vi "02_VI_DAC.vi"() -> ()   [LabVIEW 2017]
doc: "This VI illustrates how to programmatically clear different types of charts. Charts can accept a single point at a time or multiple points at a time. The charts are cleared by writing empty arrays to the History Data property node."
panel:
  out "Waveform Chart (Multiple Plots)":cluster{dbl, dbl}(graph)
  in  "Clear":bool
  out "Waveform Chart":dbl(graph)
  in  "Stop":bool
  # "Overview: Demonstrates how to programmatically clear the contents of Waveform Charts.\nInstructions:\n1. Run the VI.\n2. Click Clear to clear the contents of the charts.\n3. Click Stop to stop the VI."
  # "While the VI is running, you can right-click a chart and select Clear Chart to interactively clear the contents of the chart."
  # "Un DAC genera 2 formas de Onda! :)"
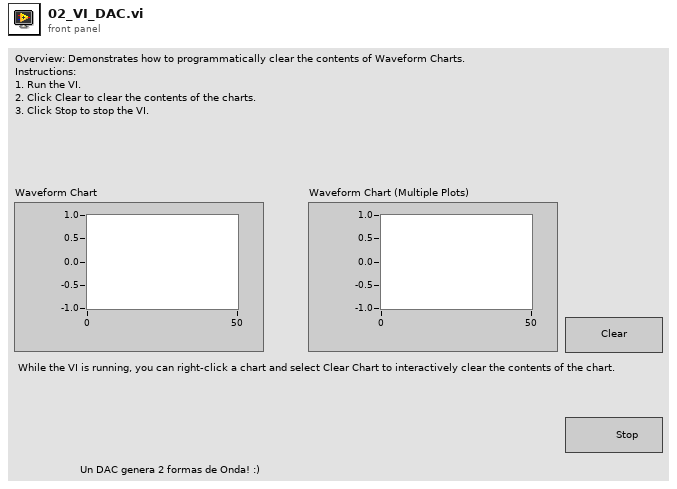
[diagram p1: front panel]
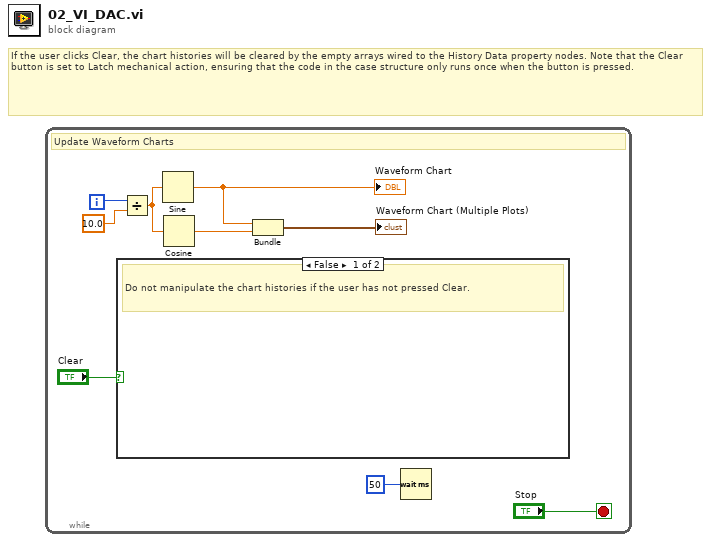
[diagram p0: block diagram]
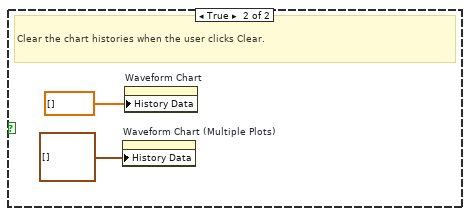
[diagram p2: hidden frame]
diagram:
  # "If the user clicks Clear, the chart histories will be cleared by the empty arrays wired to the History Data property nodes. Note that the Clear button is set to Latch mechanical action, ensuring that the code in the case structure only runs once when the button is pressed."
  n1 = while {
    i -> [w9]
    stop <- "Stop" stop-if-true
    # "Update Waveform Charts"
    n2 = case shown="False" "Clear" {
      frame False {
        # "Do not manipulate the chart histories if the user has not pressed Clear."
      }
      frame True {
        # "Clear the chart histories when the user clicks Clear."
        n3 = property on="Waveform Chart (Multiple Plots)" class="WaveformChart (strict)"("History Data"=cluster{dbl, dbl}[] []) -> ()  [unwired: 2 in, 2 out]
        n4 = property on="Waveform Chart" class="WaveformChart (strict)"("History Data"=dbl[] []) -> ()  [unwired: 2 in, 2 out]
      }
    }
    n5 = Divide(x=w9, y=10.0) -> (x/y=w8:dbl)
    n6 = Sine(x=w8) -> (sin(x)=w2:dbl)
    "Waveform Chart" <- w2
    n7 = Cosine(x=w8) -> (cos(x)=w7:dbl)
    n8 = Bundle(w2, w7) -> (→"Waveform Chart (Multiple Plots)":cluster{dbl, dbl})  [unwired: 1 in]
    n9 = Wait (ms)(milliseconds to wait=u32 50 ("millisecond multiple")) -> ()  [unwired: 1 out]
  }
